vi "Write Force Demand.vi"(10 "Force Setpoint":T1 min=-888.0 max=888.0 format="%.2f", 11 "ForceSetpoint in":refnum<class "ForceSetpoint.lvclass">) -> (3 "ForceSetpoint out":refnum<class "ForceSetpoint.lvclass">)   [LabVIEW 2013, in "ForceSetpoint.lvclass"]
uses:
  ForceSetpoint.lvclass
  Typedefs/ForceSetpoint.ctl
  ForceSetpoint.lvclass/ForceSetpoint.ctl
  Typedefs/FAMTTypedefs.lvlib
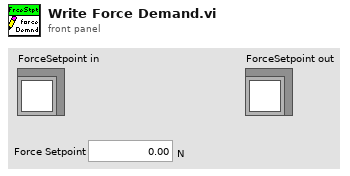
[diagram p1: front panel]
types:
  T1 = typedef "FAMTTypedefs.lvlib/ForceSetpoint.ctl" = dbl[unit]
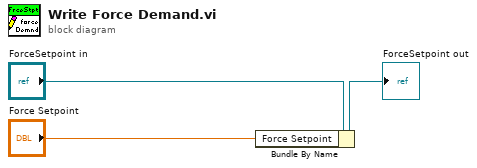
[diagram p0: block diagram]
diagram:
  n1 = Bundle By Name(cluster="ForceSetpoint in", "Force Setpoint"="Force Setpoint") -> (→"ForceSetpoint out":refnum<class "ForceSetpoint.lvclass">)
